vi "for_v0_v22.vi"() -> ()   [LabVIEW 2009]
panel:
  out "Waveform Graph":dbl[](graph)=[0.0, 0.12362590863716792, 0.24535512248077407, 0.36332004622926106, 0.47571083711452977, 0.5808031718918304, 0.6769847017710694, 0.7627797894123897, 0.8368721484658155, 0.8981250383143633, 0.9455987041886077, 0.9785647950827796, 0.9965175382696868, 0.9991814989726863, 0.986515806144185, 0.9587147795178821, 0.916204948314384, 0.8596385073398418, 0.789883310875526, 0.7080095578741987, 0.6152733727418105, 0.513097533611638, 0.4030496437817464, 0.28681808121419794, 0.16618609508385884, 0.04300444679303393, -0.08083698480075377, -0.2034381983052341, -0.32291822001593323, -0.4374439622119064, -0.545258346774607, -0.6447072626513803, -0.7342649435764969, -0.8125573766993593, -0.8783833829797784, -0.9307330459304299, -0.9688032059688466, -0.9920097826613153, -0.9999967358082196, -0.9926415278879575, -0.9700570040534724, -0.9325896608380897, -0.8808143301325396, -0.8155253599927171, -0.7377244275840832, -0.6486051712390918, -0.5495348774058578, -0.44203350345077524, -0.32775035815166476, -0.20843879765425843, -0.08592932511199664, 0.037898493279860876, 0.16114486498566233, 0.28191891814758513, 0.39836771174092883, 0.5087046637865625, 0.6112369614688756, 0.7043915326274299, 0.7867391801621942, 0.8570165090772255, 0.9141453097534555, 0.9572491000683299, 0.9856665725695978, 0.9989617403938787, 0.9969306262691764, 0.9796043919772558, 0.9472488602630078, 0.9003604365257677, 0.8396584928628675, 0.7660743313110217, 0.6807368956138382, 0.5849554507285368, 0.48019949580651805, 0.368076218827113, 0.2503058387802415, 0.12869521370345335, 0.005110119484409252, -0.11855337526675148, -0.24039799910237178, -0.3585543860764248, -0.4712097559515812, -0.5766357262563601, -0.6732148294939608, -0.7594653286701171, -0.8340639504149242, -0.895866186922294, -0.9439238552303666, -0.9774996444447237, -0.9960784277178089, -0.9993751654337899, -0.987339278346532, -0.9601554235770701, -0.9182406615650694, -0.862238057439497, -0.7930068149776356, -0.7116090945193093, -0.6192937170786801, -0.5174770046685674, -0.4077210507890664, -0.2917097544592495, -0.1712229854828543, -0.04810927730994499, 0.07574253355358546, 0.19843228647452157, 0.3180776493579683, 0.4328429977837946, 0.5409675775440859, 0.6407925185059669, 0.7307862853474564, 0.8095681746957519, 0.8759294981699033, 0.9288521263331713, 0.9675241090498167, 0.9913521325955231, 0.9999706224018354, 0.993247351778376, 0.9712854705626489, 0.9344219225734527, 0.8832222761476691, 0.8184720470714175, 0.7411646470310095, 0.6524861424810966, 0.5537970577626898, 0.44661150165145436, 0.3325739375811653, 0.2134339539384866, 0.09101942150852796, -0.032791550104701896, -0.1560994268323834, -0.27701239319366344, -0.3936753769282084, -0.5042985099065106, -0.6071845886646663, -0.7007551132582724, -0.7835745049418724, -0.8543721311211786, -0.912061799666638, -0.955758423502421, -0.984791599799224, -0.9987158954360313, -0.9973176809291077, -0.9806184079806479, -0.94887428036223, -0.9025723231824557, -0.8424229108448987, -0.7693488683340183, -0.684471313039386, -0.5890924543359805, -0.4846756148129973, -0.37282277966970634, -0.25525001872028247, -0.13376115808835443, -0.010220105525756154, 0.11347774605376376, 0.23543459809283146, 0.353779362816633, 0.4666963698566169, 0.5724532226486821, 0.6694273772270418, 0.7561310356363443, 0.8312339720420514, 0.8935839413360565, 0.9422243571244386, 0.9764089678778907, 0.995613306080252, 0.9995427347198821, 0.988136967672904, 0.9615709946256472, 0.9202523963459306, 0.8648150914928631, 0.7961096109029238, 0.7151900485662894, 0.6232978894942565, 0.5218429625940699, 0.41238181077614433, 0.29659381014407366, 0.1762554046518504, 0.05321285152564689, -0.07064610440440162, -0.19342119288395876, -0.313228772581969, -0.42823073031368747, -0.5366626817612592, -0.6368610410304885, -0.7272885437368752, -0.8065578320403944, -0.8734527397824159, -0.926946951163693, -0.9662197466980694, -0.9906685948641204, -0.9999183962709794, -0.9938272385123935, -0.9724885734168252, -0.9362297832897679, -0.8856071581452887, -0.821397360987174, -0.7445855120811328, -0.656350075031684, -0.5580447765446935, -0.45117783726642613, -0.3373888323439318, -0.21842353671694817, -0.09610714107015637, 0.02768375062767305, 0.15104991237802945, 0.27209863447893334, 0.3889727618768277, 0.4998791870315458, 0.6031163601507892, 0.6971003947263373, 0.7803893678552772, 0.8517054425256408, 0.9099544724616555, 0.9542427887469266, 0.9838909106816585, 0.998443970519014, 0.9976786921421322, 0.9816068166134568, 0.9504749220408796, 0.9047606405243412, 0.845165330223306, 0.7726033149717885, 0.6881878565290354, 0.5932140746825507, 0.4891390772468659, 0.377559604807769, 0.2601875331911011, 0.13882360950237596, 0.01532982468446124, -0.10839915354060677, -0.23046504906388943, -0.34899510114241045, -0.46217079668990607, -0.5682557702885713, -0.6656224438739162, -0.7527769973811085, -0.8283822872478106, -0.8912783611530509, -0.940500254250654, -0.9752927938636541, -0.9951221855029669, -0.999684202455144, -0.9889088532928483, -0.9629614556981103, -0.9222401001235475, -0.8673695422045798, -0.7991916176265584, -0.7187523265039294, -0.6272857854256181, -0.5261952933777384, -0.4170318020342576, -0.30147012072891755, -0.18128322117681706, -0.05831503616799799, 0.06554783043876398, 0.18840504839069752, 0.3083717163090441, 0.4236072802439881, 0.5323437718419861, 0.6329129328895512, 0.7237718100830005, 0.803526427343848, 0.8709531724941229, 0.9250175701727688, 0.9648901529750599, 0.9899591873166638, 0.9998400587794581, 0.9943811729471428, 0.9736662811987856, 0.9380131957774789, 0.8879689138478015, 0.8243012253498229, 0.7479869334037257, 0.6601968679900876, 0.5622779228291008, 0.4557323910527253, 0.3421949167062527, 0.22340741569420636, 0.10119235093876149, -0.022575228231255854, -0.14599645348305562, -0.2671777703187927, -0.38425998938849126, -0.49544681056561474, -0.5990323821628903, -0.6934274724690812, -0.7771838520774615, -0.849016512927164, -0.9078233831681786, -0.9527022353803615, -0.9829645287370384, -0.9981459727437361, -0.9980136504809862, -0.9825695920648833, -0.9520507435006151, -0.9069253314068206, -0.847885679383942, -0.7758375862393647, -0.6918864290308528, -0.5973202041383509, -0.4935897665515381]
  in  "Numarul de puncte":dbl(slide)=300.66445182724254 scale=0.0..500.0
  in  "stop":bool
  in  "Nr de perioade":dbl(knob)=5.937568360540167 scale=0.0..25.0
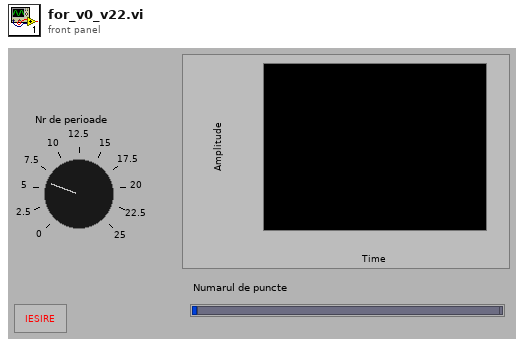
[diagram p1: front panel]
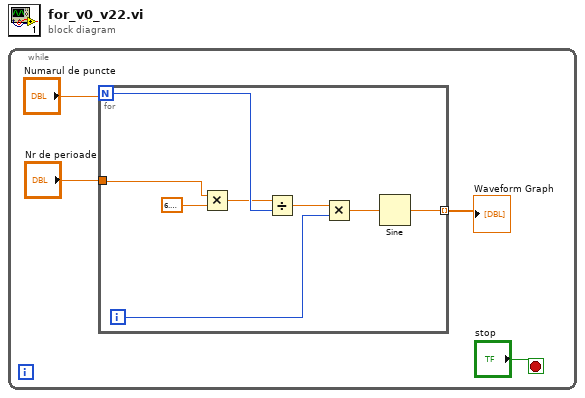
[diagram p0: block diagram]
diagram:
  n1 = while {
    stop <- "stop" stop-if-true
    n2 = for {
      N: "Numarul de puncte" -> [w11]
      tunnel: [w12] -> w1 mode=indexing
      tunnel: "Nr de perioade" -> [w6]
      i -> [w9]
      n3 = Multiply(x=w6, y=6.283185307179586) -> (x*y=w7:dbl)
      n4 = Divide(x=w7, y=w11) -> (x/y=w10:dbl)
      n5 = Multiply(x=w10, y=w9) -> (x*y=w8:dbl)
      n6 = Sine(x=w8) -> (sin(x)=w12:dbl)
    }
    "Waveform Graph" <- w1
  }
